vi "Write Set Button Names.vi"(8 "error in (no error)":errorcluster, 10 "Set Button Names":string[](array[string]), 11 "UI Populate Menu in":refnum<class "UI Populate Menu.lvclass">) -> (0 "error out":errorcluster, 3 "UI Populate Menu out":refnum<class "UI Populate Menu.lvclass">)   [LabVIEW 2011, in "UI Populate Menu.lvclass"]
uses:
  UI Populate Menu.lvclass
  UI Populate Menu.lvclass/UI Populate Menu.ctl
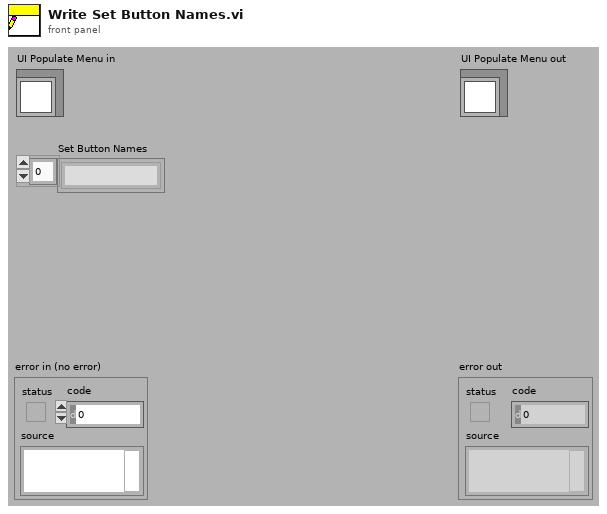
[diagram p1: front panel]
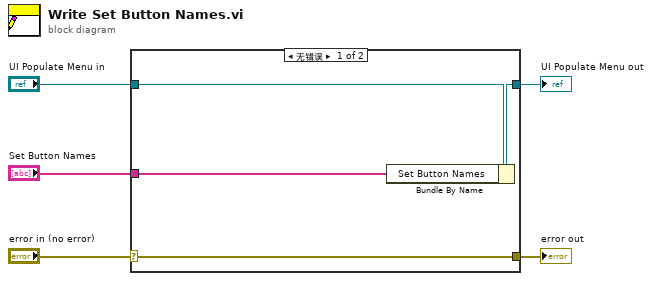
[diagram p0: block diagram]
diagram:
  n1 = case shown="无错误" "error in (no error)" {
    selector: "error in (no error)" -> [w9 w10]
    tunnel: [w9 w10] -> w4
    tunnel: [w7 w11] -> w2
    tunnel: "UI Populate Menu in" -> [w8 w11]
    tunnel: "Set Button Names" -> [w6 _]
    frame No Error {
      n2 = Bundle By Name(cluster=w8, "Set Button Names"=w6) -> (w7:refnum<class "UI Populate Menu.lvclass">)
    }
    frame Error {
    }
  }
  "error out" <- w4
  "UI Populate Menu out" <- w2
